vi "SensorDataUpdater.vi"() -> ()   [LabVIEW 2012]
uses:
  BotStatus.vi
  Concept proof/Cannon/Cannon Global Data.vi
panel:
  out "% OF RANGE":dbl(graph)
  out "Sensor Output":dbl(graph)
  out "zAvit":dbl(graph)
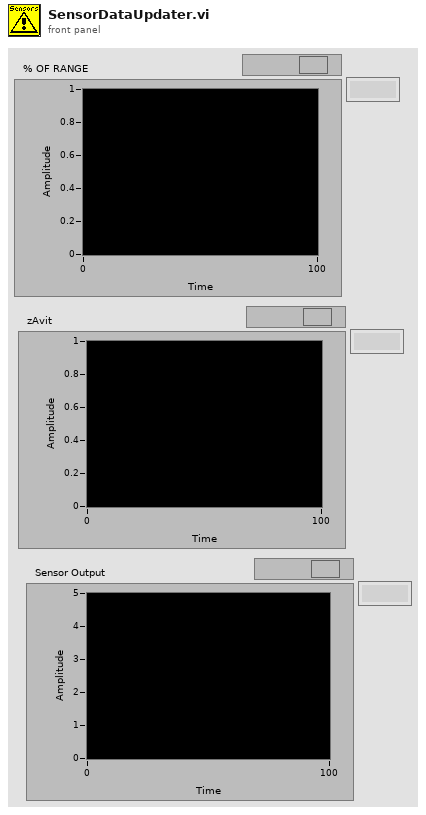
[diagram p1: front panel]
types:
  T1 = typedef "WPI_DigitalInputDevRef.ctl" = cluster{"DevStatus":errorcluster, "DIO Channel":T2, "Digital Module":T3}
  T2 = typedef "FPGA_DIOChannel.ctl" = enum8{"DIO 1", "DIO 2", "DIO 3", "DIO 4", "DIO 5", "DIO 6", "DIO 7", "DIO 8", "DIO 9", "DIO 10", "DIO 11", "DIO 12", "DIO 13", "DIO 14", "Invalid"}
  T3 = typedef "FPGA_TypedefDigitalModule.ctl" = enum16{"Digital Module 1", "Digital Module 2"}
  T4 = typedef "WPI_AnalogChannelDevRef.ctl" = cluster{"DevStatus":errorcluster, "Analog Module":T5, "Analog Channel":T6}
  T5 = typedef "FPGA_TypedefAnalogModule.ctl" = enum16{"Analog Module 1", "Analog Module 2"}
  T6 = typedef "FPGA_AIChannel.ctl" = enum8{"AI 1", "AI 2", "AI 3", "AI 4", "AI 5", "AI 6", "AI 7", "AI 8", "Invalid"}
  T7 = typedef "WPI_ServoDeviceRef.ctl" = cluster{"DeviceStatus":errorcluster, "Digital Module":T3, "PWM Channel":T8, "DeadBand":T9}
  T8 = typedef "FPGA_DIOPWMChannel.ctl" = enum8{"PWM 1", "PWM 2", "PWM 3", "PWM 4", "PWM 5", "PWM 6", "PWM 7", "PWM 8", "PWM 9", "PWM 10", "Invalid"}
  T9 = typedef "WPI_PWMDeadband.ctl" = cluster{"Name":string, "maxPositivePwm":i32, "minPositivePwm":i32, "centerPwm":i32, "maxNegativePwm":i32, "minNegativePwm":i32, "angularRange":u16}
  T10 = cluster{"Cannon Upper LS":bool, "Cannon Lower LS":bool}
  T11 = cluster{"Middle":bool, "InFlipper":bool, "Bottom":bool, "FlipperDown":bool, "Frizbee Counter":dbl}
  T12 = cluster{"RPM":dbl, "Trigger":bool, "Angle Axis":dbl, "Angle":dbl, "Throttle":dbl, "Slow Angle Change?":bool, "Angle Change?":bool}
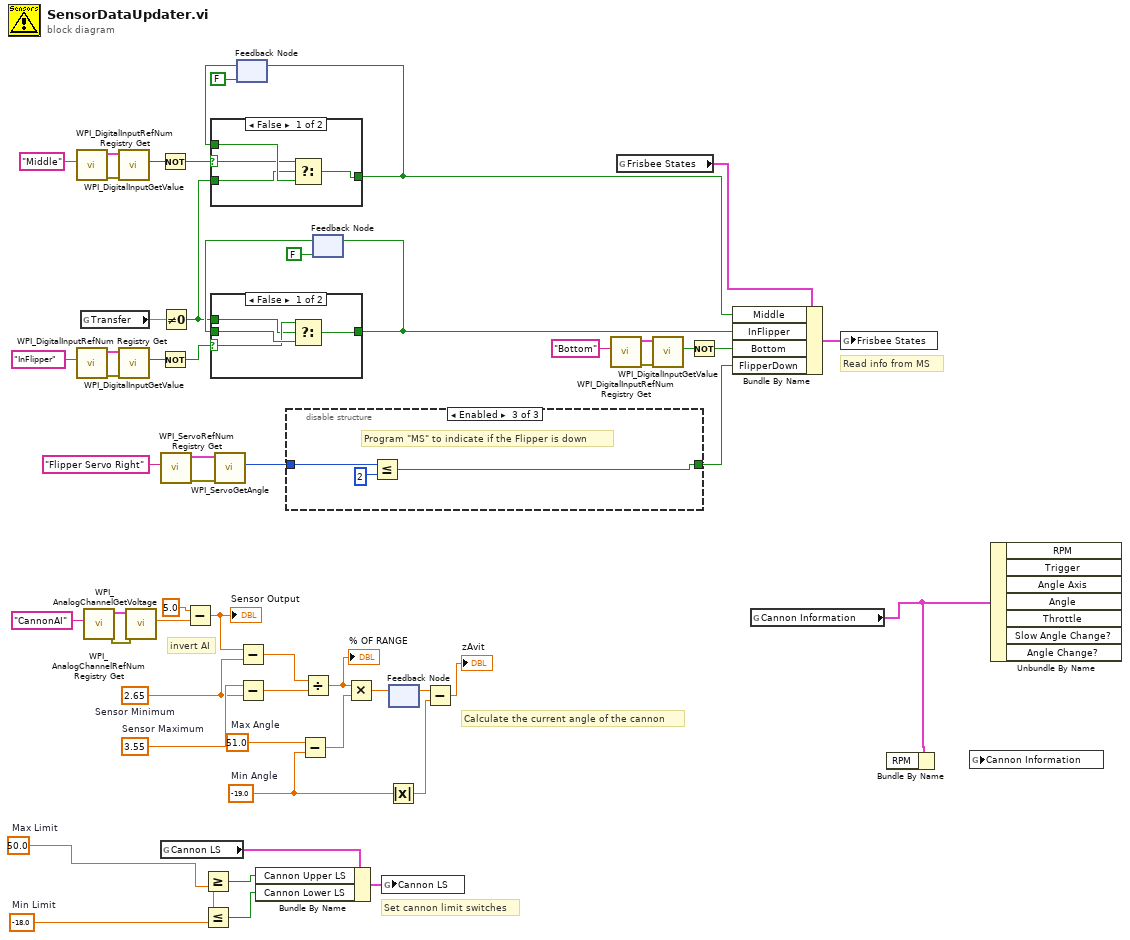
[diagram p0: block diagram]
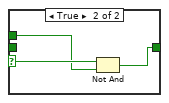
[diagram p2: hidden frame]
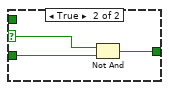
[diagram p3: hidden frame]
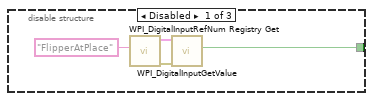
[diagram p4: hidden frame]
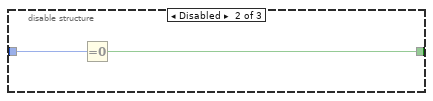
[diagram p5: hidden frame]
diagram:
  w20 = -18.0  # Min Limit
  w17 = 50.0  # Max Limit
  w29 = 2.65  # Sensor Minimum
  w30 = 3.55  # Sensor Maximum
  w22 = 51.0  # Max Angle
  w21 = -19.0  # Min Angle
  # "Read info from MS"
  # "Calculate the current angle of the cannon"
  # "Set cannon limit switches"
  # "invert AI"
  n1 = call <vilib>:"WPI_DigitalInputRefNum Registry Get.vi"("refnum name"="Middle") -> ("error out"=w48:errorcluster, "DigitalInputDevRef"=w49:T1)  [unwired: 9 in]
  n2 = call <vilib>:"WPI_DigitalInputRefNum Registry Get.vi"("refnum name"="InFlipper") -> ("error out"=w51:errorcluster, "DigitalInputDevRef"=w50:T1)  [unwired: 9 in]
  n3 = global read "BotStatus.vi" "Transfer"() -> (w11:dbl)
  n4 = call <vilib>:"WPI_AnalogChannelRefNum Registry Get.vi"("refnum name"="CannonAI") -> ("error out"=w43:errorcluster, "AIDeviceRef"=w44:T4)  [unwired: 9 in]
  n5 = call <vilib>:"WPI_DigitalInputGetValue.vi"("error in (no error)"=w48, "DigitalInputDevRef"=w49) -> ("Value"=w47:bool)  [unwired: 7 in, 2 out]
  n6 = call <vilib>:"WPI_DigitalInputGetValue.vi"("error in (no error)"=w51, "DigitalInputDevRef"=w50) -> ("Value"=w46:bool)  [unwired: 7 in, 2 out]
  n7 = call <vilib>:"WPI_AnalogChannelGetVoltage.vi"("error in (no error)"=w43, "AIDeviceRef"=w44) -> ("Voltage"=w25:dbl)  [unwired: 7 in, 2 out]
  n8 = Not(x=w47) -> (.not. x?=w7:bool)
  n9 = Not(x=w46) -> (.not. x?=w3:bool)
  n10 = Not Equal To 0?(x=w11) -> (x != 0?=w2:bool)
  n11 = call <vilib>:"WPI_ServoRefNum Registry Get.vi"("refnum name"="Flipper Servo Right") -> ("error out"=w42:errorcluster, "ServoDeviceRef"=w41:T7)  [unwired: 9 in]
  n12 = global read "BotStatus.vi" "Cannon LS"() -> (w38:T10)
  n13 = Subtract(x=5.0, y=w25) -> (x-y=w24:dbl)
  "Sensor Output" <- w24
  n14 = Less Or Equal?(y=w20) -> (x=w16:dbl, x <= y?=w35:bool)
  n15 = Greater Or Equal?(x=w16, y=w17) -> (x >= y?=w36:bool)
  n16 = call <vilib>:"WPI_ServoGetAngle.vi"("ServoDeviceRef"=w41, "error in (no error)"=w42) -> ("Angle"=w39:u16)  [unwired: 6 in, 2 out]
  n17 = feedback #1(FALSE) -> (w10:bool)
  n18 = case shown="False" w7 {
    selector: w7 -> [w58 w63]
    tunnel: [w60 w62] -> w8
    tunnel: w10 -> [w59 _]
    tunnel: w2 -> [w57 w61]
    frame False {
      n19 = Select(t=w58, s=w57, f=w59) -> (s? t:f=w60:bool)
    }
    frame True {
      n20 = Not And(1:w61, 2:w63) -> (0:w62:bool)
    }
  }
  n21 = feedback-in #1(w8) -> ()
  n22 = Subtract(x=w24, y=w29) -> (x-y=w27:dbl)
  n23 = Subtract(x=w30, y=w29) -> (x-y=w28:dbl)
  n24 = Bundle By Name(cluster=w38, "Cannon Upper LS"=w36, "Cannon Lower LS"=w35) -> (w37:T10)
  n25 = disable-structure shown="Enabled" {
    disable-tunnel: [w64 w69 w71] -> w12
    disable-tunnel: w39 -> [_ w68 w70]
    frame Disabled {
      n26 = call <vilib>:"WPI_DigitalInputRefNum Registry Get.vi"("refnum name"="FlipperAtPlace") -> ("error out"=w66:errorcluster, "DigitalInputDevRef"=w67:T1)  [unwired: 9 in]
      n27 = call <vilib>:"WPI_DigitalInputGetValue.vi"("error in (no error)"=w66, "DigitalInputDevRef"=w67) -> ("Value"=w64:bool)  [unwired: 7 in, 2 out]
    }
    frame Disabled {
      n28 = Equal To 0?(x=w68) -> (x = 0?=w69:bool)
    }
    frame Enabled {
      # "Program \"MS\" to indicate if the Flipper is down"
      n29 = Less Or Equal?(x=w70, y=2) -> (x <= y?=w71:bool)
    }
  }
  n30 = Subtract(x=w22, y=w21) -> (x-y=w34:dbl)
  n31 = Divide(x=w27, y=w28) -> (x/y=w33:dbl)
  "% OF RANGE" <- w33
  n32 = feedback #2(FALSE) -> (w5:bool)
  n33 = case shown="False" w3 {
    selector: w3 -> [w74 w79]
    tunnel: [w76 w78] -> w4
    tunnel: w5 -> [w75 _]
    tunnel: w2 -> [w73 w77]
    frame False {
      n34 = Select(t=w74, s=w73, f=w75) -> (s? t:f=w76:bool)
    }
    frame True {
      n35 = Not And(1:w77, 2:w79) -> (0:w78:bool)
    }
  }
  n36 = feedback-in #2(w4) -> ()
  n37 = Multiply(x=w33, y=w34) -> (x*y=w32:dbl)
  n38 = global write "BotStatus.vi" "Cannon LS"(w37) -> ()
  n39 = Absolute Value(x=w21) -> (abs(x)=w23:dbl)
  n40 = feedback #3() -> (w31:dbl)  [unwired: 1 in]
  n41 = feedback-in #3(w32) -> ()
  n42 = Subtract(x=w31, y=w23) -> (x-y=→"zAvit":dbl)
  n43 = call <vilib>:"WPI_DigitalInputRefNum Registry Get.vi"("refnum name"="Bottom") -> ("error out"=w53:errorcluster, "DigitalInputDevRef"=w52:T1)  [unwired: 9 in]
  n44 = global read "BotStatus.vi" "Frisbee States"() -> (w15:T11)
  n45 = call <vilib>:"WPI_DigitalInputGetValue.vi"("error in (no error)"=w53, "DigitalInputDevRef"=w52) -> ("Value"=w18:bool)  [unwired: 7 in, 2 out]
  n46 = Not(x=w18) -> (.not. x?=w13:bool)
  n47 = Bundle By Name(cluster=w15, "Middle"=w8, "InFlipper"=w4, "Bottom"=w13, "FlipperDown"=w12) -> (w14:T11)
  n48 = global read "Cannon Global Data.vi" "Cannon Information"() -> (w1:T12)
  n49 = global write "BotStatus.vi" "Frisbee States"(w14) -> ()
  n50 = Bundle By Name(cluster=w1) -> ()  [unwired: 1 in, 1 out]
  n51 = global read "Cannon Global Data.vi" "Cannon Information"() -> ()  [unwired: 1 in]
  n52 = Unbundle By Name(w1) -> ()  [unwired: 7 out]
